vi "BestY.vi"(0 "Utilities in":refnum<class "Utilities.lvclass">, 1 "Game":refnum<class "Game.lvclass">, 2 "inimigos":bool, 3 "error in (no error)":errorcluster) -> (4 "Eclipse":bool, 6 "Utilities out":refnum<class "Utilities.lvclass">, 7 "Best y":dbl, 8 "Gap kick":dbl, 9 "error out":errorcluster)   [LabVIEW 2018, in "Utilities.lvclass"]
uses:
  Utilities.lvclass
  Game_class/Game.lvclass
  segment.ctl
  Vision_class/Old vision/SSL Detection Frame Simple Estimator Cameras VelCmd Folder/Core/AI Ball.ctl
  pos.ctl
  Game_class/Game.lvclass/Game.ctl
  Team_class/Team.lvclass/Team.ctl
  Object_class/Object.lvclass/Object.ctl
  Object_class/Read x.vi
  Object_class/Read y.vi
  <vilib>/Analysis/baseanly.llb/Real Dot Product.vi
  Game_class/Read BallRef.vi
  Game_class/Read FieldRef.vi
  Game_class/Read EnemyRef.vi
  Game_class/Read AllyRef.vi
  Team_class/Read RobotRef.vi
  Ally_class/Ally.lvclass
  Enemy_class/Enemy.lvclass
  Ball_class/Ball.lvclass
  Robot_class/Robot.lvclass
  Field_class/Field.lvclass
  <vilib>/Analysis/NI_AALBase.lvlib
panel:
  out "Vetor de gaps \ncorreto":T1[](array[typedef])
  out "Gap Coord":dbl[](array[numeric])
  in  "Ball false":dbl[](array[numeric])
  in  "Best y para varredura?":bool
  out "Vetor de gaps":T1[](array[typedef])
  in  "Maior intervalo":bool
  in  "eclipse angle eps":dbl=0.035 format="%#_13g"
  out "pilha output (merged)":T1[](array[typedef])
  out "Vetor de segmentos ordenado":T1[](array[typedef])
  out "Vetor de segmentos (sombras)":T1[](array[typedef])
types:
  T1 = typedef "Utilities.lvclass/segment.ctl" = cluster{"up":dbl, "down":dbl}
  T2 = typedef "pos.ctl" = cluster{"x":dbl, "y":dbl}
  T3 = typedef "AI Ball.ctl" = cluster{"x":dbl, "y":dbl, "timestamp":timestamp, "Vel_x":dbl, "Vel_y":dbl, "Pos Bola Est":dbl[], "Valid":bool}
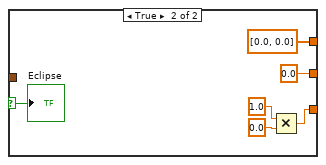
[diagram p4: hidden frame]
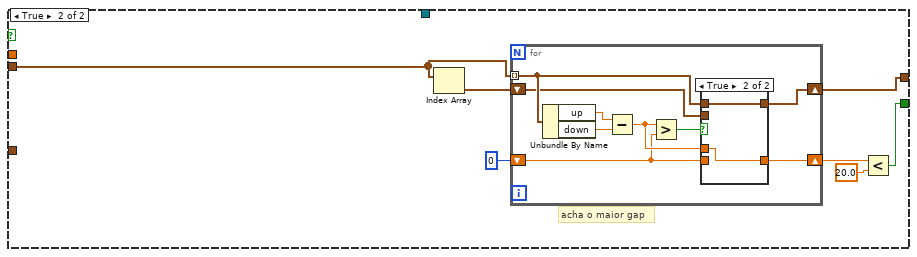
[diagram p7: hidden frame]
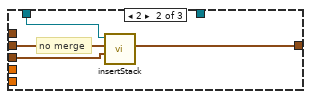
[diagram p9: hidden frame]
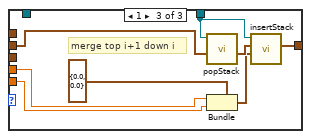
[diagram p10: hidden frame]
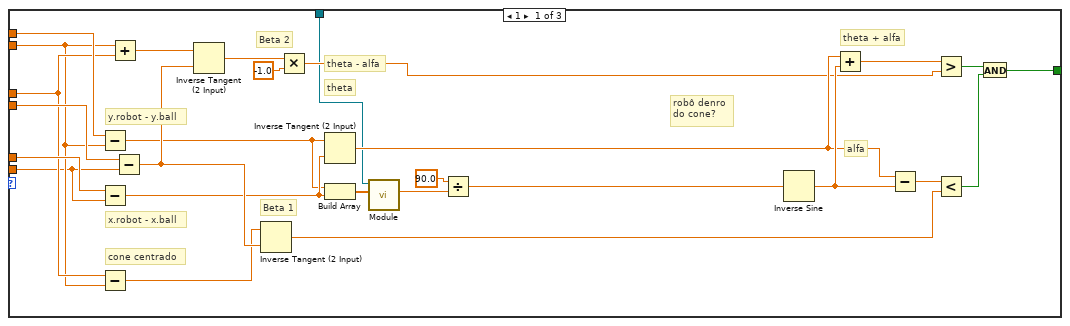
[diagram p12: hidden frame]
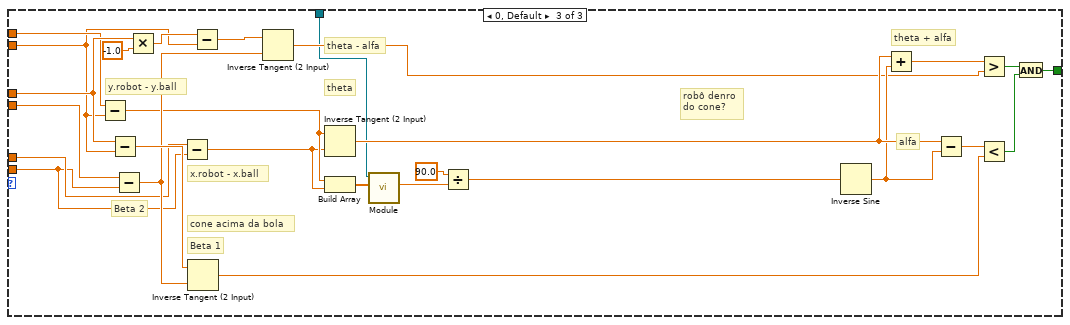
[diagram p13: hidden frame]
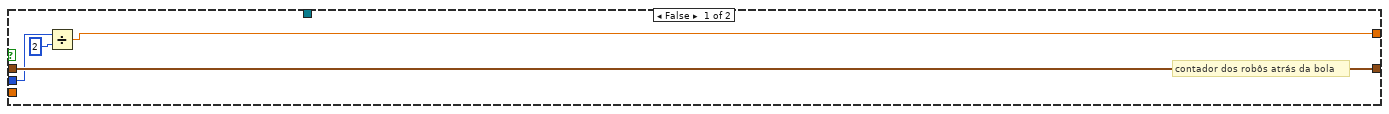
[diagram p14: hidden frame]
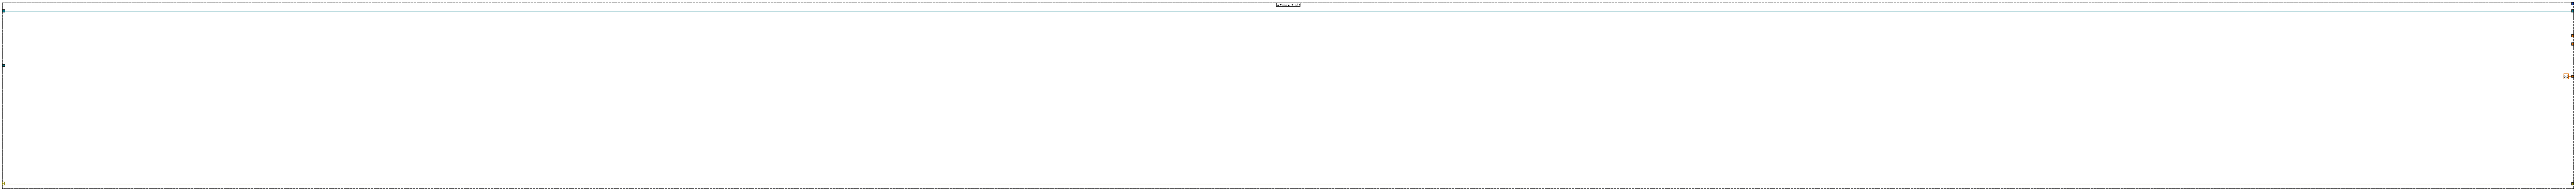
[diagram p16: hidden frame]
diagram:
  # "Gap kick is now a value from 0 to 1\n0 -> goal not free\n1 - > goal totally free"
  n1 = case shown="No Error" "error in (no error)" {
    selector: "error in (no error)" -> [w63 w426]
    tunnel: [w63 w426] -> w9
    tunnel: [w12 w425] -> w7
    tunnel: "Utilities in" -> [w12 w425]
    tunnel: "Game" -> [w27 _]
    tunnel: [w23 _] -> w5
    tunnel: [w22 _] -> w1
    tunnel: [w21 0.0] -> w4
    tunnel: [w11 _] -> w2
    frame No Error {
      w40 = T3 {"x"=0.0, "y"=0.0, "timestamp"=timestamp(0 s since 1904-01-01), "Vel_x"=0.0, "Vel_y"=0.0, "Pos Bola Est"=[], "Valid"=FALSE} ("element")
      # "goal_width/2"
      # "field_length/2"
      # "balls"
      # "vetor de gaps"
      # "upper"
      n2 = property class="Game"(reference=w27) -> ("BallRef"=w26:refnum<class "Ball.lvclass">, "FieldRef"=w19:refnum<class "Field.lvclass">, "EnemyRef"=w16:refnum<class "Enemy.lvclass">, "AllyRef"=w14:refnum<class "Ally.lvclass">)  [unwired: 1 in, 2 out]
      n3 = property class="Enemy"(reference=w16) -> ("RobotRef"=w15:refnum<class "Robot.lvclass">[])  [unwired: 1 in, 2 out]
      n4 = property class="Ally"(reference=w14) -> ("RobotRef"=w13:refnum<class "Robot.lvclass">[])  [unwired: 1 in, 2 out]
      n5 = property class="Ball"(reference=w26) -> ("x"=w25:dbl, "y"=w24:dbl)  [unwired: 1 in, 2 out]
      n6 = property class="Field"(reference=w19) -> ("field_length"=w17:i32, "goal_width"=w11:i32)  [unwired: 1 in, 2 out]
      n7 = Bundle By Name(cluster=T2 {"x"=0.0, "y"=0.0} ("pos"), "x"=w25, "y"=w24) -> (w18:T2)
      n8 = Select(t=w15, s="inimigos", f=w13) -> (s? t:f=w45:refnum<class "Robot.lvclass">[])
      n9 = Index Array(array="Ball false") -> (element #1=w43:dbl, element #2=w42:dbl)  [unwired: 2 in]
      n10 = Bundle By Name(cluster=w40, "x"=w43, "y"=w42) -> ()  [unwired: 1 out]
      n11 = case shown="False" "Best y para varredura?" {
        tunnel: [w118 w119] -> w39
        tunnel: w18 -> [w118 w119]
        tunnel: w40 -> [_ _]
        frame False {
        }
        frame True {
        }
      }
      n12 = Divide(x=w11, y=u32 2 ("x")) -> (x/y=w32:dbl)
      n13 = for {
        shift-right: [w267] -> w48
        shift-left: T1[] [] -> [w266]
        tunnel: w17 -> [w244]
        tunnel: w32 -> [w246]
        tunnel: w32 -> [w264]
        shift-right: [w263] -> w46
        shift-left: _ -> [_]
        tunnel: w45 -> [w236] mode=indexing
        tunnel: "inimigos" -> [w261]
        tunnel: w39 -> [w240]
        tunnel: w12 -> [w233]
        tunnel: w12 -> [w232]
        # "y ball"
        # "x ball"
        # "y.robot"
        # "x.robot"
        # "field_length/2"
        # "goal_width/2"
        # "y ball"
        # "x ball"
        n14 = property class="Robot"(reference=w236) -> ("x"=w235:dbl, "y"=w234:dbl)  [unwired: 1 in, 2 out]
        n15 = Unbundle By Name(w240) -> ("x"=w239:dbl, "y"=w237:dbl)
        n16 = Divide(x=w244, y=2.0) -> (x/y=w243:dbl)
        n17 = Multiply(x=w246, y=-1.0) -> (x*y=w250:dbl)
        n18 = Greater?(x=w237, y=w246) -> (0:w249:bool)
        n19 = Less?(x=w237, y=w250) -> (x < y?=w248:bool)
        n20 = Absolute Value(x=w239) -> (abs(x)=w259:dbl)
        n21 = Absolute Value(x=w235) -> (abs(x)=w265:dbl)
        n22 = Multiply(x=w235, y=-1.0) -> (x*y=w260:dbl)
        n23 = Greater?(x=w265, y=w259) -> (0:w258:bool)
        n24 = Select(t=w235, s=w261, f=w260) -> (s? t:f=w241:dbl)
        n25 = Select(t=1, s=w249, f=0) -> (s? t:f=w256:i32)
        n26 = Select(t=0, s=w248, f=1) -> (s? t:f=w257:i32)
        n27 = Add(x=w256, y=w257) -> (x+y=w247:i32)
        n28 = case shown="2" w247 {
          tunnel: w246 -> [w271 w298 w347]
          tunnel: w243 -> [w292 w318 w349]
          tunnel: w241 -> [w279 w305 w342]
          tunnel: w234 -> [w278 w306 w343]
          tunnel: [w280 w307 w333] -> w238
          tunnel: w239 -> [w269 w296 w325]
          tunnel: w237 -> [w270 w297 w326]
          tunnel: w233 -> [w268 w295 w324]
          frame 1 {
            # "robô denro\ndo cone?"
            # "cone centrado"
            # "theta - alfa"
            # "theta + alfa"
            # "theta"
            # "alfa"
            # "x.robot - x.ball"
            # "y.robot - y.ball"
            # "Beta 2"
            # "Beta 1"
            n29 = Subtract(x=w278, y=w270) -> (x-y=w281:dbl)
            n30 = Subtract(x=w279, y=w269) -> (x-y=w282:dbl)
            n31 = Subtract(x=w271, y=w270) -> (x-y=w293:dbl)
            n32 = Add(x=w270, y=w271) -> (x+y=w291:dbl)
            n33 = Subtract(x=w292, y=w269) -> (x-y=w294:dbl)
            n34 = Inverse Tangent (2 Input)(1:w294, 2:w291) -> (0:w290:dbl)
            n35 = Inverse Tangent (2 Input)(1:w294, 2:w293) -> (0:w274:dbl)
            n36 = Multiply(x=w290, y=-1.0) -> (x*y=w276:dbl)
            n37 = Inverse Tangent (2 Input)(1:w282, 2:w281) -> (0:w287:dbl)
            n38 = Build Array(w281, w282) -> (w283:dbl[])
            n39 = call-dynamic "Module.vi"("2D vector"=w283, "Utilities in"=w268) -> ("Modulo"=w284:dbl)  [unwired: 7 in, 2 out]
            n40 = Divide(x=90.0, y=w284) -> (x/y=w285:dbl)
            n41 = Inverse Sine(1:w285) -> (0:w288:dbl)
            n42 = Add(x=w287, y=w288) -> (x+y=w277:dbl)
            n43 = Subtract(x=w287, y=w288) -> (x-y=w275:dbl)
            n44 = Greater?(x=w277, y=w276) -> (0:w272:bool)
            n45 = Less?(x=w275, y=w274) -> (x < y?=w273:bool)
            n46 = And(x=w272, y=w273) -> (x .and. y?=w280:bool)
          }
          frame 2 {
            # "robô denro\ndo cone?"
            # "cone abaixo da bola"
            # "theta - alfa"
            # "theta + alfa"
            # "theta"
            # "alfa"
            # "x.robot - x.ball"
            # "y.robot - y.ball"
            # "Beta 2"
            # "Beta 1"
            n47 = Add(x=w297, y=w298) -> (x+y=w321:dbl)
            n48 = Subtract(x=w297, y=w298) -> (x-y=w320:dbl)
            n49 = Subtract(x=w318, y=w296) -> (x-y=w319:dbl)
            n50 = Inverse Tangent (2 Input)(1:w319, 2:w320) -> (0:w316:dbl)
            n51 = Inverse Tangent (2 Input)(1:w319, 2:w321) -> (0:w322:dbl)
            n52 = Subtract(x=w306, y=w297) -> (x-y=w308:dbl)
            n53 = Multiply(x=w322, y=-1.0) -> (x*y=w303:dbl)
            n54 = Subtract(x=w305, y=w296) -> (x-y=w309:dbl)
            n55 = Inverse Tangent (2 Input)(1:w309, 2:w308) -> (0:w314:dbl)
            n56 = Build Array(w308, w309) -> (w310:dbl[])
            n57 = call-dynamic "Module.vi"("2D vector"=w310, "Utilities in"=w295) -> ("Modulo"=w311:dbl)  [unwired: 7 in, 2 out]
            n58 = Multiply(x=w316, y=-1.0) -> (x*y=w301:dbl)
            n59 = Divide(x=90.0, y=w311) -> (x/y=w312:dbl)
            n60 = Inverse Sine(1:w312) -> (0:w315:dbl)
            n61 = Add(x=w314, y=w315) -> (x+y=w304:dbl)
            n62 = Subtract(x=w314, y=w315) -> (x-y=w302:dbl)
            n63 = Less?(x=w302, y=w301) -> (x < y?=w300:bool)
            n64 = Greater?(x=w304, y=w303) -> (0:w299:bool)
            n65 = And(x=w299, y=w300) -> (x .and. y?=w307:bool)
          }
          frame 0, Default {
            # "robô denro\ndo cone?"
            # "cone acima da bola"
            # "theta - alfa"
            # "theta + alfa"
            # "theta"
            # "alfa"
            # "x.robot - x.ball"
            # "y.robot - y.ball"
            # "Beta 2"
            # "Beta 1"
            n66 = Subtract(x=w343, y=w326) -> (x-y=w341:dbl)
            n67 = Subtract(x=w347, y=w326) -> (x-y=w350:dbl)
            n68 = Subtract(x=w349, y=w325) -> (x-y=w344:dbl)
            n69 = Multiply(x=w347, y=-1.0) -> (x*y=w346:dbl)
            n70 = Subtract(x=w342, y=w325) -> (x-y=w340:dbl)
            n71 = Inverse Tangent (2 Input)(1:w344, 2:w350) -> (0:w328:dbl)
            n72 = Subtract(x=w346, y=w326) -> (x-y=w345:dbl)
            n73 = Inverse Tangent (2 Input)(1:w344, 2:w345) -> (0:w331:dbl)
            n74 = Inverse Tangent (2 Input)(1:w340, 2:w341) -> (0:w335:dbl)
            n75 = Build Array(w341, w340) -> (w339:dbl[])
            n76 = call-dynamic "Module.vi"("2D vector"=w339, "Utilities in"=w324) -> ("Modulo"=w338:dbl)  [unwired: 7 in, 2 out]
            n77 = Divide(x=90.0, y=w338) -> (x/y=w337:dbl)
            n78 = Inverse Sine(1:w337) -> (0:w334:dbl)
            n79 = Add(x=w335, y=w334) -> (x+y=w332:dbl)
            n80 = Subtract(x=w335, y=w334) -> (x-y=w329:dbl)
            n81 = Greater?(x=w332, y=w331) -> (0:w330:bool)
            n82 = Less?(x=w329, y=w328) -> (x < y?=w327:bool)
            n83 = And(x=w330, y=w327) -> (x .and. y?=w333:bool)
          }
        }
        n84 = And(x=w258, y=w238) -> (x .and. y?=w242:bool)
        n85 = case shown="True" w242 {
          tunnel: [w354 w362] -> w267
          tunnel: w266 -> [w354 w364]
          tunnel: w244 -> [w353 w369]
          tunnel: w246 -> [_ w368]
          tunnel: w264 -> [_ w361]
          tunnel: [w351 w360] -> w263
          tunnel: w234 -> [_ w359]
          tunnel: w241 -> [_ w358]
          tunnel: w239 -> [_ w356]
          tunnel: w237 -> [_ w357]
          tunnel: w232 -> [_ w355]
          frame False {
            # "contador dos robôs atrás da bola"
            n86 = Divide(x=w353, y=u32 2) -> (x/y=w351:dbl)
          }
          frame True {
            n87 = flat-sequence {
              tunnel: w359 -> [w405]
              tunnel: w369 -> [w401]
              tunnel: w368 -> [w386]
              tunnel: [w376] -> w367
              tunnel: [w375] -> w366
              tunnel: [w387] -> w365
              tunnel: w364 -> [w380]
              tunnel: [w380] -> w363
              tunnel: [w374] -> w360
              tunnel: w358 -> [w373]
              tunnel: w357 -> [w371]
              tunnel: w356 -> [w372]
              tunnel: w355 -> [w370]
              tunnel: w367 -> [w409]
              tunnel: w366 -> [w408]
              tunnel: w365 -> [w410]
              tunnel: w363 -> [w411]
              tunnel: [w407] -> w362
              tunnel: w361 -> [w406]
              frame #0 {
                # "theta - alfa"
                # "alfa + theta"
                # "theta"
                # "alfa"
                # "x.robot - x.ball"
                # "y.robot - y.ball"
                n88 = Subtract(x=w405, y=w371) -> (x-y=w385:dbl)
                n89 = Subtract(x=w373, y=w372) -> (x-y=w384:dbl)
                n90 = Inverse Tangent (2 Input)(1:w384, 2:w385) -> (0:w383:dbl)
                n91 = Build Array(w385, w384) -> (w404:dbl[])
                n92 = call-dynamic "Module.vi"("2D vector"=w404, "Utilities in"=w370) -> ("Modulo"=w402:dbl)  [unwired: 7 in, 2 out]
                n93 = Divide(x=90.0, y=w402) -> (x/y=w382:dbl)
                n94 = Inverse Sine(1:w382) -> (0:w381:dbl)
                n95 = Add(x=w383, y=w381) -> (x+y=w399:dbl)
                n96 = Subtract(x=w383, y=w381) -> (x-y=w397:dbl)
                n97 = Divide(x=w401, y=u32 2 ("x")) -> (x/y=w374:dbl)
                n98 = Subtract(x=w374, y=w372) -> (x-y=w377:dbl)
                n99 = Tangent(1:w397) -> (0:w396:dbl)
                n100 = Multiply(x=w396, y=w377) -> (x*y=w378:dbl)
                n101 = Tangent(1:w399) -> (0:w398:dbl)
                n102 = Multiply(x=w398, y=w377) -> (x*y=w379:dbl)
                n103 = Add(x=w378, y=w371) -> (x+y=w375:dbl)
                n104 = Multiply(x=w386, y=-1.0) -> (x*y=w392:dbl)
                n105 = Add(x=w379, y=w371) -> (x+y=w376:dbl)
                n106 = Greater?(x=w375, y=w386) -> (0:w394:bool)
                n107 = Less?(x=w375, y=w392) -> (x < y?=w390:bool)
                n108 = Greater?(x=w376, y=w386) -> (0:w395:bool)
                n109 = Less?(x=w376, y=w392) -> (x < y?=w391:bool)
                n110 = And(x=w395, y=w394) -> (x .and. y?=w389:bool)
                n111 = And(x=w391, y=w390) -> (x .and. y?=w388:bool)
                n112 = Or(x=w389, y=w388) -> (x .or. y?=w387:bool)
              }
              frame #1 {
                # "goal_width/2"
                n113 = case shown="False" w410 {
                  tunnel: [w420 w423] -> w407
                  tunnel: w411 -> [w419 w423]
                  tunnel: w409 -> [w418 _]
                  tunnel: w408 -> [w416 _]
                  tunnel: w406 -> [w415 _]
                  frame False {
                    n114 = Max & Min(x=w418, y=w415) -> (min(x,y)=w417:dbl)  [unwired: 1 out]
                    n115 = Multiply(x=w415, y=-1.0) -> (x*y=w413:dbl)
                    n116 = Max & Min(x=w416, y=w413) -> (max(x,y)=w412:dbl)  [unwired: 1 out]
                    n117 = Bundle(cluster=T1 {"up"=0.0, "down"=0.0} ("segment 2"), "up"=w417, "down"=w412) -> (w421:T1)
                    n118 = Insert Into Array(array=w419, new element=w421) -> (w420:T1[])  [unwired: 1 in]
                  }
                  frame True {
                  }
                }
              }
            }
          }
        }
      }
      "Vetor de segmentos (sombras)" <- w48
      n119 = Multiply(x=w32, y=-1.0) -> (x*y=w49:dbl)
      n120 = Sort 1D Array(array=w48) -> (sorted array=w60:T1[])
      "Vetor de segmentos ordenado" <- w60
      n121 = Index Array(array=w60) -> (element=w59:T1)  [unwired: 1 in]
      n122 = call-dynamic "insertStack.vi"("novo elemento"=w59, "pilha input"=T1[] [], "Utilities in"=w12) -> ("pilha output"=w57:T1[])  [unwired: 5 in, 2 out]
      n123 = for {
        shift-right: [w190] -> w56
        shift-left: w57 -> [w192]
        tunnel: w60 -> [w191] mode=indexing
        tunnel: w12 -> [w189]
        tunnel: w12 -> [w188]
        tunnel: w12 -> [w187]
        i -> [w193]
        n124 = case shown="Default" w193 {
          tunnel: w192 -> [w200 w231]
          tunnel: w191 -> [w203 _]
          tunnel: [w201 w231] -> w190
          tunnel: w189 -> [w196 _]
          tunnel: w188 -> [w195 _]
          tunnel: w187 -> [w194 _]
          frame Default {
            # "pilha"
            # "i+1"
            # "i"
            # "i+1"
            # "i"
            n125 = Unbundle By Name(w203) -> ("down"=w198:dbl, "up"=w205:dbl)
            n126 = call-dynamic "topStack.vi"("pilha input"=w200, "Utilities in"=w194) -> ("top"=w202:T1)  [unwired: 7 in, 2 out]
            n127 = Unbundle By Name(w202) -> ("up"=w199:dbl, "down"=w204:dbl)
            n128 = Greater Or Equal?(x=w198, y=w199) -> (x >= y?=w197:bool)
            n129 = Less?(x=w198, y=w204) -> (x < y?=w207:bool)
            n130 = Select(t=1, s=w197, f=0) -> (s? t:f=w209:i32)
            n131 = Select(t=0, s=w207, f=1) -> (s? t:f=w208:i32)
            n132 = Add(x=w209, y=w208) -> (x+y=w206:i32)
            n133 = case shown="0, Default" w206 {
              tunnel: w205 -> [_ _ w229]
              tunnel: w204 -> [_ _ w228]
              tunnel: w202 -> [_ _ _]
              tunnel: w203 -> [w215 w221 _]
              tunnel: [w218 w220 w224] -> w201
              tunnel: w200 -> [w217 w222 w227]
              tunnel: w196 -> [w214 w219 _]
              tunnel: w195 -> [_ _ w223]
              frame 0, Default {
                # "merge:  i+1"
                n134 = call-dynamic "popStack.vi"("pilha input"=w217, "Utilities in"=w214) -> ("pilha output"=w216:T1[])  [unwired: 7 in, 2 out]
                n135 = call-dynamic "insertStack.vi"("novo elemento"=w215, "pilha input"=w216, "Utilities in"=w214) -> ("pilha output"=w218:T1[])  [unwired: 5 in, 2 out]
              }
              frame 2 {
                # "no merge"
                n136 = call-dynamic "insertStack.vi"("novo elemento"=w221, "pilha input"=w222, "Utilities in"=w219) -> ("pilha output"=w220:T1[])  [unwired: 5 in, 2 out]
              }
              frame 1 {
                # "merge top i+1 down i"
                n137 = call-dynamic "popStack.vi"("pilha input"=w227, "Utilities in"=w223) -> ("pilha output"=w226:T1[])  [unwired: 7 in, 2 out]
                n138 = Bundle(cluster=T1 {"up"=0.0, "down"=0.0} ("segment 2"), "up"=w229, "down"=w228) -> (w225:T1)
                n139 = call-dynamic "insertStack.vi"("novo elemento"=w225, "pilha input"=w226, "Utilities in"=w223) -> ("pilha output"=w224:T1[])  [unwired: 5 in, 2 out]
              }
            }
          }
          frame 0 {
          }
        }
      }
      "pilha output (merged)" <- w56
      n140 = Reverse 1D Array(array=w56) -> (reversed array=w55:T1[])
      n141 = for {
        tunnel: w55 -> [w186] mode=indexing
        shift-right: [w180] -> w52
        shift-left: T1[] [] -> [w182]
        shift-right: [w181] -> w51
        shift-left: w32 -> [w183]
        n142 = Unbundle By Name(w186) -> ("up"=w179:dbl, "down"=w181:dbl)
        n143 = Bundle(cluster=T1 {"up"=0.0, "down"=0.0} ("segment 2"), "up"=w183, "down"=w179) -> (w185:T1)
        n144 = Insert Into Array(array=w182, new element=w185) -> (w180:T1[])  [unwired: 1 in]
      }
      n145 = Bundle(cluster=T1 {"up"=0.0, "down"=0.0} ("segment 2"), "up"=w51, "down"=w49) -> (w54:T1)
      n146 = Insert Into Array(array=w52, new element=w54) -> (w33:T1[])  [unwired: 1 in]
      n147 = Array Size(array=w33) -> (size(s)=w35:i32)
      n148 = Decrement(x=w35) -> (x-1=w34:i32)
      n149 = for {
        N: w34 -> [_]
        shift-right: [w82] -> w31
        shift-left: w33 -> [w84]
        i -> [w83]
        n150 = Increment(x=w83) -> (x+1=w92:i32)
        n151 = Index Array(array=w84, index=w83) -> (element=w85:T1)
        n152 = Index Array(array=w84, index=w92) -> (element=w91:T1)
        n153 = Unbundle By Name(w85) -> ("up"=w87:dbl, "down"=w90:dbl)
        n154 = Unbundle By Name(w91) -> ("up"=w89:dbl, "down"=w86:dbl)
        n155 = Equal?(x=w90, y=w89) -> (x = y?=w88:bool)
        n156 = case shown="True" w88 {
          tunnel: w87 -> [_ w102]
          tunnel: w86 -> [_ w101]
          tunnel: w85 -> [_ w100]
          tunnel: w84 -> [w93 w98]
          tunnel: w83 -> [_ w95]
          tunnel: [w93 w94] -> w82
          frame False {
          }
          frame True {
            n157 = Bundle By Name(cluster=w100, "up"=w102, "down"=w101) -> (w96:T1)
            n158 = Delete From Array(array=w98, length=2, index=w95) -> (array with subset deleted=w97:T1[])  [unwired: 1 out]
            n159 = Insert Into Array(array=w97, index=w95, new element=w96) -> (w94:T1[])
          }
        }
      }
      "Vetor de gaps" <- w31
      n160 = for {
        tunnel: w32 -> [w73]
        tunnel: w31 -> [w66] mode=indexing
        shift-right: [w68] -> w28
        shift-left: T1[] [] -> [w67]
        n161 = Unbundle By Name(w66) -> ("up"=w65:dbl, "down"=w64:dbl)
        n162 = Multiply(x=w73, y=-1.0) -> (x*y=w72:dbl)
        n163 = Greater?(x=w65, y=w73) -> (0:w70:bool)
        n164 = Less?(x=w64, y=w72) -> (x < y?=w69:bool)
        n165 = Or(x=w70, y=w69) -> (x .or. y?=w71:bool)
        n166 = case shown="False" w71 {
          tunnel: [w75 w78] -> w68
          tunnel: w67 -> [w75 w79]
          tunnel: w65 -> [_ w76]
          tunnel: w64 -> [_ w77]
          frame True {
          }
          frame False {
            n167 = Bundle(cluster=T1 {"up"=0.0, "down"=0.0} ("segment 2"), "up"=w76, "down"=w77) -> (w80:T1)
            n168 = Insert Into Array(array=w79, new element=w80) -> (w78:T1[])  [unwired: 1 in]
          }
        }
      }
      "Vetor de gaps \ncorreto" <- w28
      n169 = case shown="False" "Maior intervalo" {
        tunnel: [w123 w162] -> w36
        tunnel: [w122 w160] -> w37
        tunnel: w28 -> [w129 w161]
        tunnel: w39 -> [w121 _]
        tunnel: w46 -> [w126 _]
        tunnel: w12 -> [w120 _]
        frame False {
          # "acha o maior ângulo"
          n170 = Index Array(array=w129) -> (element=w130:T1)  [unwired: 1 in]
          n171 = Unbundle By Name(w121) -> ("x"=w128:dbl, "y"=w127:dbl)
          n172 = for {
            tunnel: w129 -> [w152] mode=indexing
            shift-right: [w153] -> w125
            shift-left: 0 -> [w135]
            shift-right: [w151] -> w122
            shift-left: w130 -> [w150]
            tunnel: w128 -> [w134]
            tunnel: w127 -> [w133]
            tunnel: w126 -> [w149]
            tunnel: w120 -> [w132]
            # "theta"
            # "cos (theta)"
            # "vetor bola-down"
            # "vetor bola-up"
            n173 = Unbundle By Name(w152) -> ("up"=w148:dbl, "down"=w145:dbl)
            n174 = Subtract(x=w149, y=w134) -> (x-y=w146:dbl)
            n175 = Subtract(x=w148, y=w133) -> (x-y=w147:dbl)
            n176 = Subtract(x=w145, y=w133) -> (x-y=w144:dbl)
            n177 = Build Array(w146, w144) -> (w142:dbl[])
            n178 = Build Array(w146, w147) -> (w143:dbl[])
            n179 = call-dynamic "Module.vi"("2D vector"=w143, "Utilities in"=w132) -> ("Modulo"=w141:dbl)  [unwired: 7 in, 2 out]
            n180 = call-poly <vilib>:"Dot Product.vi"("Y Vector"=w142, "X Vector"=w143) -> ("X * Y"=w139:dbl)  [unwired: 1 out]
            n181 = call-dynamic "Module.vi"("2D vector"=w142, "Utilities in"=w132) -> ("Modulo"=w140:dbl)  [unwired: 7 in, 2 out]
            n182 = Multiply(x=w141, y=w140) -> (x*y=w138:dbl)
            n183 = Divide(x=w139, y=w138) -> (x/y=w137:dbl)
            n184 = Inverse Cosine(1:w137) -> (0:w136:dbl)
            n185 = Greater?(x=w136, y=w135) -> (0:w154:bool)
            n186 = case shown="True" w154 {
              tunnel: w136 -> [_ w158]
              tunnel: [w155 w158] -> w153
              tunnel: w152 -> [_ w157]
              tunnel: [w156 w157] -> w151
              tunnel: w150 -> [w156 _]
              tunnel: w135 -> [w155 _]
              frame False {
              }
              frame True {
              }
            }
          }
          n187 = Less?(x=w125, y="eclipse angle eps") -> (x < y?=w123:bool)
        }
        frame True {
          # "acha o maior gap"
          n188 = Index Array(array=w161) -> (element=w164:T1)  [unwired: 1 in]
          n189 = for {
            tunnel: w161 -> [w169] mode=indexing
            shift-right: [w170] -> w163
            shift-left: 0 -> [w167]
            shift-right: [w168] -> w160
            shift-left: w164 -> [w166]
            n190 = Unbundle By Name(w169) -> ("up"=w174:dbl, "down"=w173:dbl)
            n191 = Subtract(x=w174, y=w173) -> (x-y=w171:dbl)
            n192 = Greater?(x=w171, y=w167) -> (0:w172:bool)
            n193 = case shown="True" w172 {
              tunnel: w171 -> [_ w178]
              tunnel: [w176 w178] -> w170
              tunnel: w169 -> [_ w177]
              tunnel: [w175 w177] -> w168
              tunnel: w167 -> [w176 _]
              tunnel: w166 -> [w175 _]
              frame False {
              }
              frame True {
              }
            }
          }
          n194 = Less?(x=w163, y=20.0) -> (x < y?=w162:bool)
        }
      }
      n195 = case shown="False" w36 {
        selector: w36 -> [_ w117]
        tunnel: w37 -> [w109 _]
        tunnel: [w108 w114] -> w21
        tunnel: [w106 0.0] -> w22
        tunnel: [w103 dbl[] [0.0, 0.0] ("Gap Coord")] -> w23
        frame False {
          n196 = Unbundle By Name(w109) -> ("up"=w105:dbl, "down"=w104:dbl)
          n197 = Subtract(x=w105, y=w104) -> (x-y=w107:dbl)
          n198 = Add(x=w105, y=w104) -> (x+y=w110:dbl)
          n199 = Build Array(w105, w104) -> (w103:dbl[])
          n200 = Absolute Value(x=w107) -> (abs(x)=w106:dbl)
          n201 = Divide(x=w110, y=2.0) -> (x/y=w108:dbl)
        }
        frame True {
          n202 = Multiply(x=1.0, y=0.0) -> (x*y=w114:dbl)
          "Eclipse" <- w117
        }
      }
    }
    frame Error {
    }
  }
  "error out" <- w9
  "Utilities out" <- w7
  "Gap Coord" <- w5
  "Best y" <- w4
  n203 = Divide(x=w1, y=w2) -> (x/y=→"Gap kick":dbl)
